vi "SplitSignals-Complete.vi"(0 "Filename":path=path "E:/LabVIEW/Data/Test Data/Subj-Austin_Trial-1_Condition-None.lvm", 11 "Error In":errorcluster) -> (4 "Filename Out":path=path "E:/LabVIEW/Data/Test Data/Subj-Austin_Trial-1_Condition-None.lvm" caption="Filename", 8 "Audio":dynamicdata(graph), 10 "Pressure":dynamicdata(graph), 15 "Error Out":errorcluster)   [LabVIEW 2013]
panel:
  out "Signals":dynamicdata(graph)
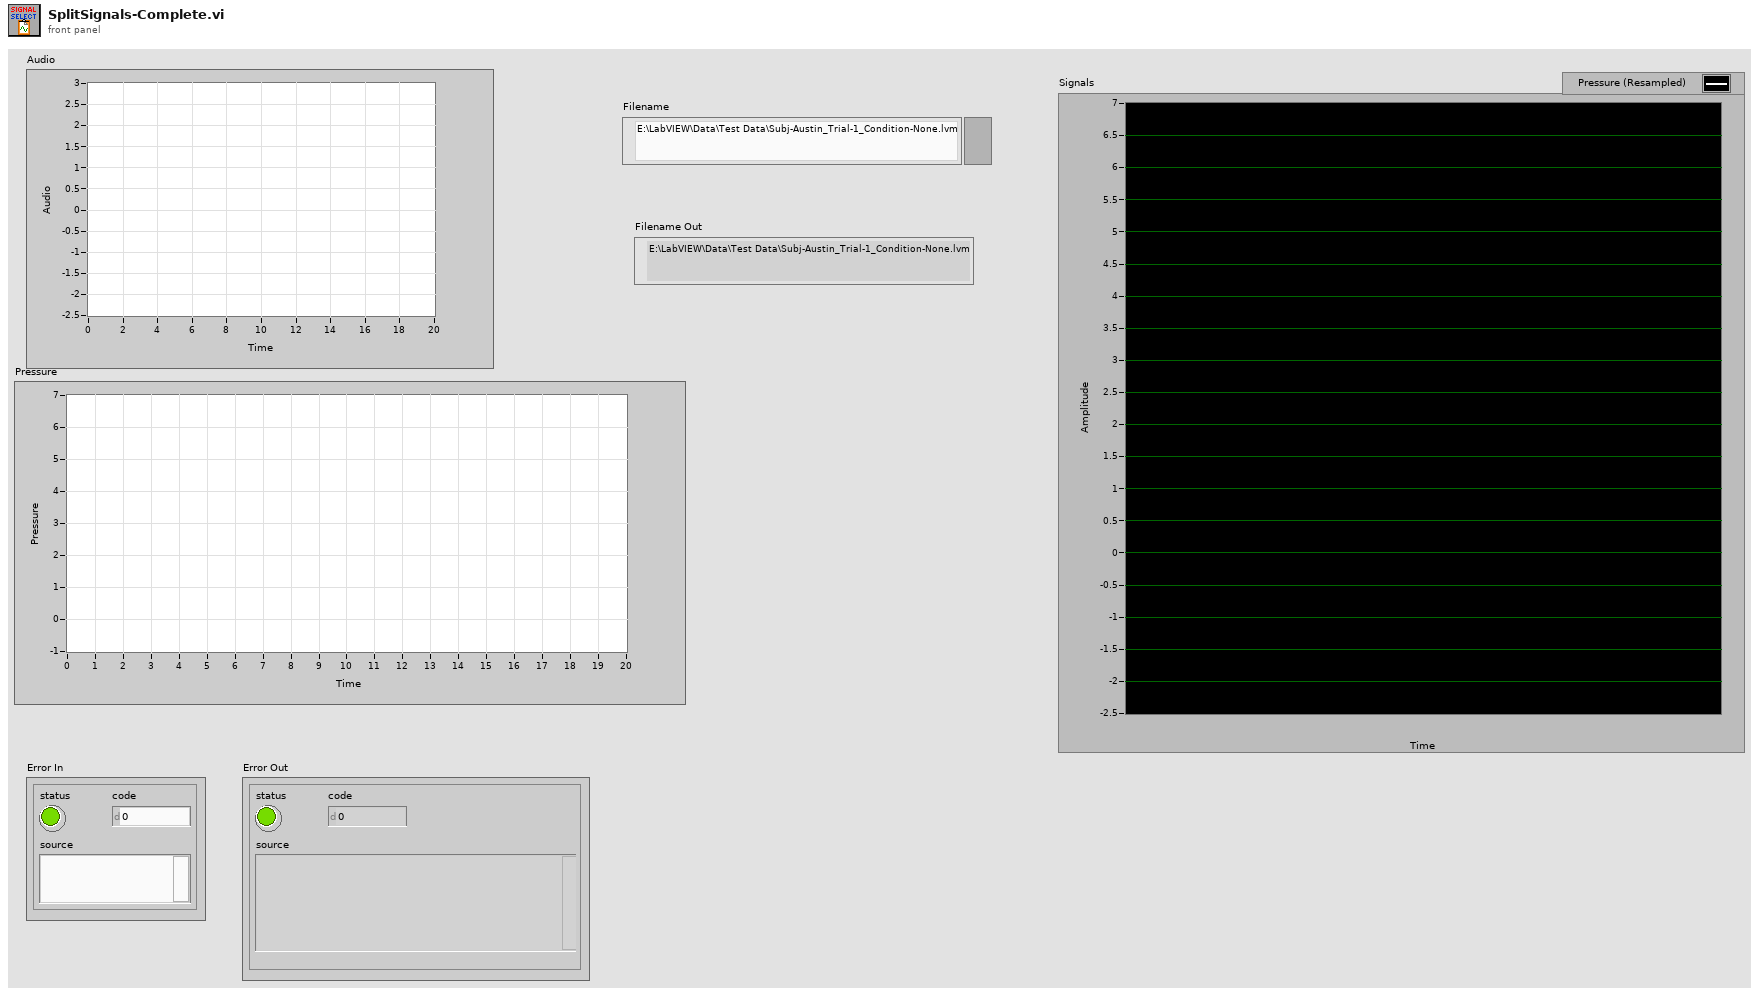
[diagram p1: front panel]
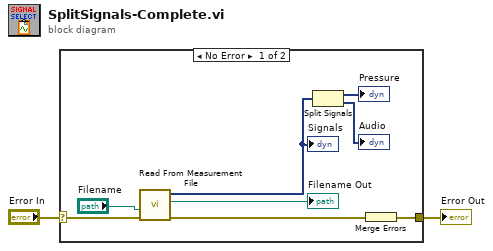
[diagram p0: block diagram]
diagram:
  n1 = case shown="No Error" "Error In" {
    selector: "Error In" -> [w8 w11]
    tunnel: [w10 w11] -> w1
    frame No Error {
      n2 = call "Read From Measurement File"("error in (no error)"=w8, "Filename"="Filename") -> ("error out"=w7:errorcluster, "Filename Out"=→"Filename Out":path, "Signals"=w6:dynamicdata)  [unwired: 4 in, 3 out]
      "Signals" <- w6
      n3 = Split Signals(w6) -> (→"Pressure":dynamicdata, →"Audio":dynamicdata)  [unwired: 2 in]
      n4 = Merge Errors(w7) -> (w10:errorcluster)
    }
    frame Error {
    }
  }
  "Error Out" <- w1
